vi "sub_SDR_mimo_SNR_Pilots.vi"(11 "Decimated Array":cdb[](array[numeric])) -> (3 "SNR (dB)":dbl)   [LabVIEW 2012]
uses:
  <vilib>/Analysis/NI_AALBase.lvlib
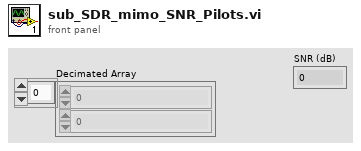
[diagram p1: front panel]
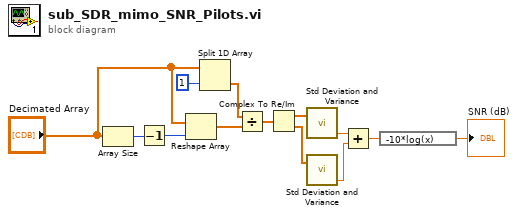
[diagram p0: block diagram]
diagram:
  n1 = Array Size(array="Decimated Array") -> (size(s)=w7:i32)
  n2 = Decrement(x=w7) -> (x-1=w6:i32)
  n3 = Reshape Array("Decimated Array", w6) -> (w3:cdb[])
  n4 = Split 1D Array(array="Decimated Array", index=1) -> (second subarray=w2:cdb[])  [unwired: 1 out]
  n5 = Divide(x=w2, y=w3) -> (x/y=w4:cdb[])
  n6 = Complex To Re/Im(x + iy=w4) -> (x=w12:dbl[], y=w11:dbl[])
  n7 = call <vilib>:"Std Deviation and Variance.vi"("X"=w12) -> ("variance"=w10:dbl)  [unwired: 1 in, 2 out]
  n8 = call <vilib>:"Std Deviation and Variance.vi"("X"=w11) -> ("variance"=w9:dbl)  [unwired: 1 in, 2 out]
  n9 = Add(x=w10, y=w9) -> (x+y=w1:dbl)
  n10 = expression code="-10*log(x)"(w1) -> (→"SNR (dB)":dbl)
